vi "Select Channels to Publish.vi"(8 "error in (no error)":errorcluster, 11 "Node Ptr":u64 format="%.0x") -> (0 "error out":errorcluster, 3 "Controller Ref out":T1 format="%.0x")   [LabVIEW 2026, in "WebPage Addon System Explorer.lvlib"]
uses:
  WebPage Addon System Explorer.lvlib
  <vilib>/NI VeriStand/Custom Device API/Custom Device Item Ref.ctl
  <vilib>/NI VeriStand/Custom Device API/Set Item Property (Dependent Node Pointer).vi
  <vilib>/NI VeriStand/Custom Device API/Custom Device API.lvlib
  <vilib>/NI VeriStand/Custom Device Tools/Custom Device Utility Library/Custom Device Utility Library.lvlib
panel:
  in  "Tag":string
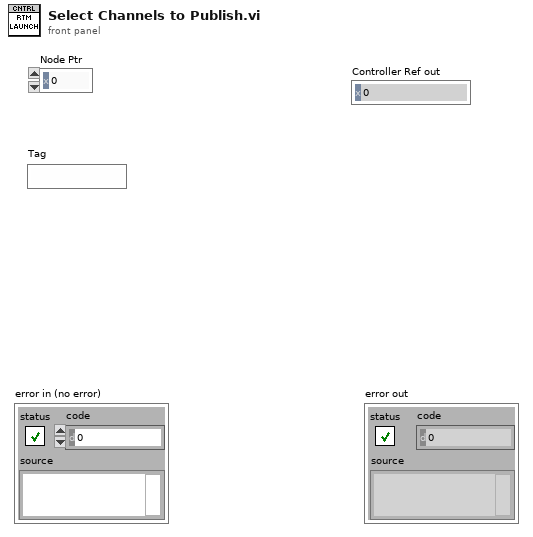
[diagram p1: front panel]
types:
  T1 = typedef "Custom Device API.lvlib/Custom Device Item Ref.ctl" = u64
  T2 = typedef "Custom Device API.lvlib/Custom Device Pointer.ctl" = refnum<k24>
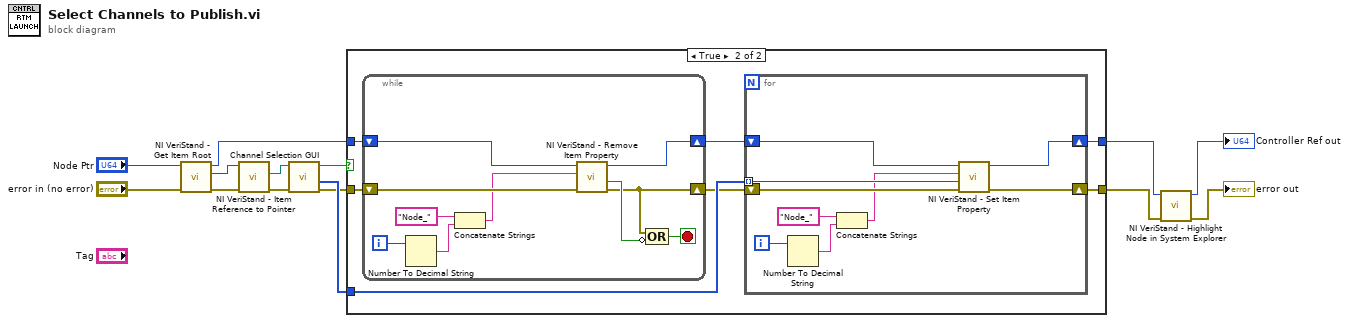
[diagram p0: block diagram]
diagram:
  n1 = call <vilib>:"NI VeriStand - Get Item Root.vi"("error in (no error)"="error in (no error)", "Item Ref in"="Node Ptr") -> ("error out"=w11:errorcluster, "Root Ref out"=w12:T1, "Item Ref out"=w7:T1)  [unwired: 6 in, 1 out]
  n2 = call <vilib>:"NI VeriStand - Item Reference to Pointer.vi"("error in (no error)"=w11, "Item Ref in"=w12) -> ("error out"=w10:errorcluster, "Node Pointer"=w9:T2)  [unwired: 6 in, 2 out]
  n3 = call "Channel Selection GUI.vi"("error in (no error)"=w10, "StartNode"=w9) -> ("error out"=w6:errorcluster, "IDs"=w8:u64[], "Apply"=w5:bool)  [unwired: 7 in]
  n4 = case shown="True" w5 {
    tunnel: [w15 w23] -> w1
    tunnel: w8 -> [_ w22]
    tunnel: [w16 w21] -> w4
    tunnel: w7 -> [w15 w20]
    tunnel: w6 -> [w16 w18]
    frame False {
    }
    frame True {
      n5 = while {
        shift-right: [w32] -> w19
        shift-left: w20 -> [w33]
        shift-right: [w24] -> w17
        shift-left: w18 -> [w31]
        i -> [w29]
        stop <- w25 stop-if-true
        n6 = Number To Decimal String(number=w29) -> (decimal integer string=w28:string)  [unwired: 1 in]
        n7 = Concatenate Strings("Node_", w28) -> (w27:string)
        n8 = call <vilib>:"NI VeriStand - Remove Item Property.vi"("error in (no error)"=w31, "Property Name"=w27, "Item Ref in"=w33) -> ("error out"=w24:errorcluster, "Removed"=w26:bool, "Item Ref out"=w32:T1)  [unwired: 6 in]
        n9 = Compound Arithmetic op=OR(w24, invert w26) -> (w25:bool)
      }
      n10 = for {
        tunnel: w22 -> [w40] mode=indexing
        shift-right: [w41] -> w23
        shift-left: w19 -> [w42]
        shift-right: [w38] -> w21
        shift-left: w17 -> [w39]
        i -> [w36]
        n11 = Number To Decimal String(number=w36) -> (decimal integer string=w35:string)  [unwired: 1 in]
        n12 = Concatenate Strings("Node_", w35) -> (w34:string)
        n13 = call-poly <vilib>:"NI VeriStand - Set Item Property.vi"("error in (no error)"=w39, "Dependent Node Ref"=w40, "Property Name"=w34, "Item Ref in"=w42) -> ("error out"=w38:errorcluster, "Item Ref out"=w41:T1)  [unwired: 5 in, 1 out]
      }
    }
  }
  n14 = call <vilib>:"NI VeriStand - Highlight Node in System Explorer.vi"("error in (no error)"=w4, "Item Ref in"=w1) -> ("error out"=→"error out":errorcluster, "Node Ptr dup"=→"Controller Ref out":T1)  [unwired: 8 in]
